vi "UsrProfiles-Save user profile-All values.vi"(8 "error in":errorcluster, 11 "Which file? (User profile.ini)":T1=enum."Loaded User profile.ini") -> (0 "error out":errorcluster)   [LabVIEW 2017]
uses:
  Typedefs/Which path.ctl
  Typedefs/Save-Load enum.ctl
  Typedefs/HW config states enum.ctl
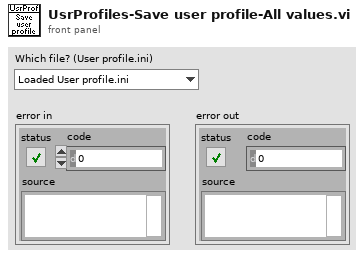
[diagram p1: front panel]
types:
  T1 = typedef "Which path.ctl" = enum16{"Configuration Files", "Calibration Files", "Images", "Setup.ini", "Loaded User profile.ini", "User's-Previous session.ini", "New user profile.ini", "Selected User profile.ini", "User profiles folder", "Power meter scaling.txt", "FOV Cal.ini"}
  T2 = typedef "HW config states enum.ctl" = enum16{"Load from file", "Save to file", "Write all", "Read all", "Write XY stage settings", "Write DAQ FPGA settings", "Write Control FPGA settings", "Write Phys Channels", "Clear", "Compare from file"}
  T3 = typedef "Save-Load enum.ctl" = enum16{"Save to file", "Load from file", "Compare from file"}
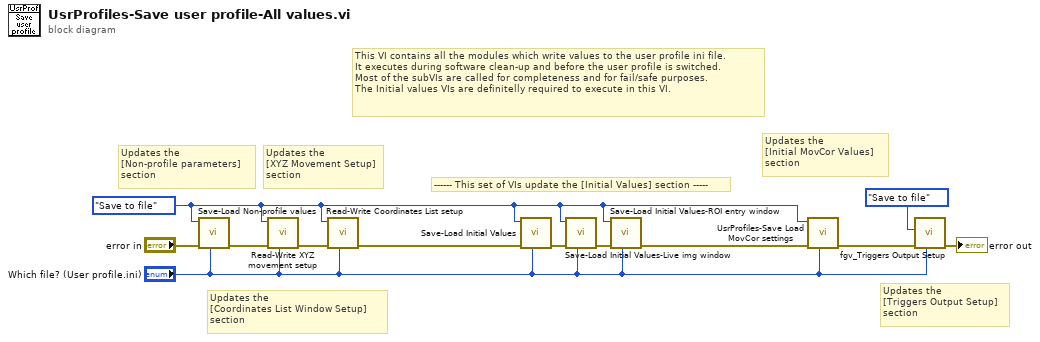
[diagram p0: block diagram]
diagram:
  w2 = Save-Load_enum."Save to file" ("Function")
  # "Updates the\n[Initial MovCor Values]\nsection"
  # "------ This set of VIs update the [Initial Values] section -----"
  # "Updates the\n[Non-profile parameters]\nsection"
  # "Updates the\n[Triggers Output Setup]\nsection"
  # "Updates the\n[Coordinates List Window Setup]\nsection"
  # "Updates the\n[XYZ Movement Setup]\nsection"
  # "This VI contains all the modules which write values to the user profile ini file.\nIt executes during software clean-up and before the user profile is switched.\nMost of the subVIs are called for completeness and for fail/safe purposes.\nThe Initial values VIs are definitelly required to execute in this VI."
  n1 = call "Save-Load Non-profile values.vi"("Which file? (User profile.ini)"="Which file? (User profile.ini)", "error in"="error in", "Function"=w2) -> ("error out"=w7:errorcluster)  [unwired: 8 in]
  n2 = call "Read-Write XYZ movement setup.vi"("Which file? (User profile.ini)"="Which file? (User profile.ini)", "error in"=w7, "Function"=w2) -> ("error out"=w8:errorcluster)  [unwired: 8 in]
  n3 = call "Read-Write Coordinates List setup.vi"("Which file?"="Which file? (User profile.ini)", "error in"=w8, "Function"=w2) -> ("error out"=w5:errorcluster)  [unwired: 8 in]
  n4 = call "Save-Load Initial Values.vi"("Which file? (User profile.ini)"="Which file? (User profile.ini)", "error in"=w5, "Function"=w2) -> ("error out"=w11:errorcluster)  [unwired: 8 in]
  n5 = call "Save-Load Initial Values-Live img window.vi"("Which file? (User profile.ini)"="Which file? (User profile.ini)", "error in"=w11, "Function"=w2) -> ("error out"=w12:errorcluster)  [unwired: 8 in]
  n6 = call "Save-Load Initial Values-ROI entry window.vi"("Which file? (User profile.ini)"="Which file? (User profile.ini)", "error in"=w12, "Function"=w2) -> ("error out"=w1:errorcluster)  [unwired: 8 in]
  n7 = call "UsrProfiles-Save Load MovCor settings.vi"("Which file? (User profile.ini)"="Which file? (User profile.ini)", "error in (no error)"=w1, "Function"=w2) -> ("error out"=w4:errorcluster)  [unwired: 8 in]
  n8 = call "fgv_Triggers Output Setup.vi"("Which file? (User profile.ini)"="Which file? (User profile.ini)", "error in (no error)"=w4, "Function"=HW_config_states_enum."Save to file") -> ("error out"=→"error out":errorcluster)  [unwired: 6 in, 2 out]
